vi "Write DAQmx Digitizer.lvclass.vi"(8 "error in (no error)":errorcluster, 10 "DAQmx Digitizer.lvclass":refnum<class "DAQmx Digitizer.lvclass">, 11 "DAQmx Recorder in":refnum<class "DAQmx Recorder.lvclass">) -> (0 "error out":errorcluster, 3 "DAQmx Recorder out":refnum<class "DAQmx Recorder.lvclass">)   [LabVIEW 2015]
uses:
  DAQmx Recorder.lvclass
  NHMFL_Core/Libraries/NI-DAQ/DAQmx Digitizer/DAQmx Digitizer.lvclass
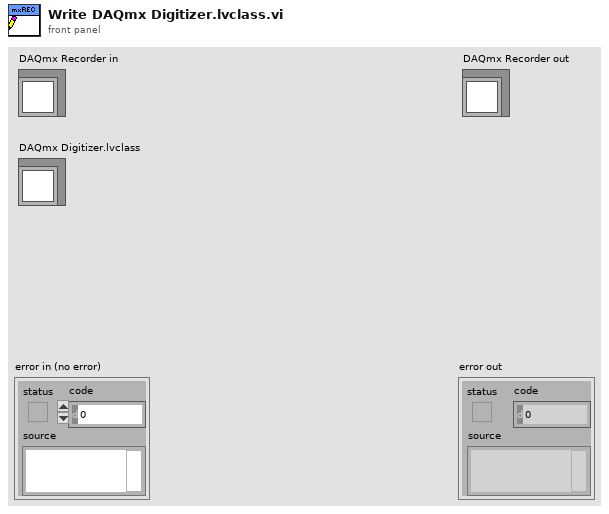
[diagram p1: front panel]
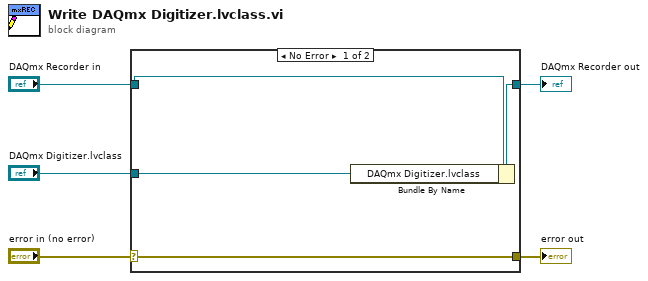
[diagram p0: block diagram]
diagram:
  n1 = case shown="No Error" "error in (no error)" {
    selector: "error in (no error)" -> [w9 w10]
    tunnel: [w9 w10] -> w4
    tunnel: [w7 w11] -> w2
    tunnel: "DAQmx Recorder in" -> [w8 w11]
    tunnel: "DAQmx Digitizer.lvclass" -> [w6 _]
    frame No Error {
      n2 = Bundle By Name(cluster=w8, "DAQmx Digitizer.lvclass"=w6) -> (w7:refnum<class "DAQmx Recorder.lvclass">)
    }
    frame Error {
    }
  }
  "error out" <- w4
  "DAQmx Recorder out" <- w2
